vi "CreateAPSxObject.vi"(0 "PGIType":enum16{"APSX_PGI_TYPE_1", "APSX_PGI_TYPE_2"}(ring), 5 "DeviceNumber":i32, 7 "PGIChannel":i32, 9 "AsicName":string, 11 "error in (no error)":errorcluster caption="错误输入（无错误）") -> (4 "hASIC":i32, 10 "Message":string, 15 "error out":errorcluster caption="错误输出")   [LabVIEW 2018]
uses:
  APSx.dll/APSx.dll
panel:
  in  "hASIC IN":i32
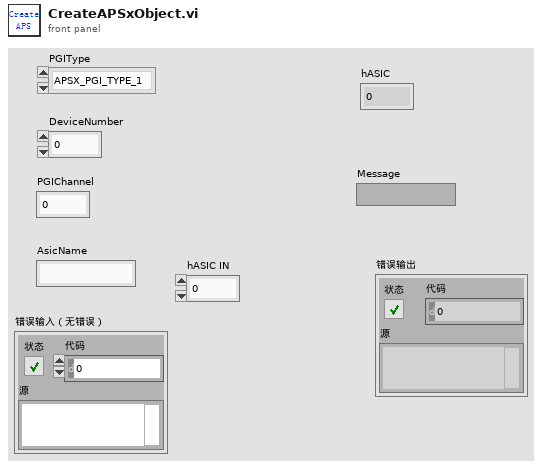
[diagram p1: front panel]
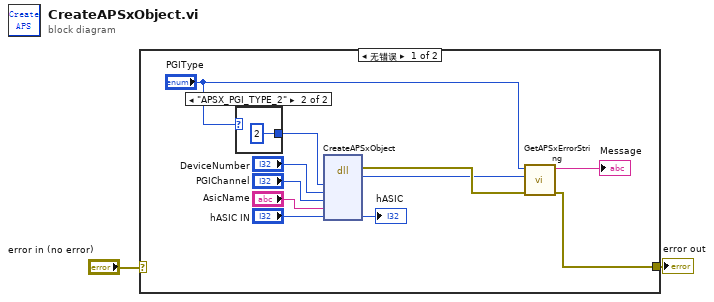
[diagram p0: block diagram]
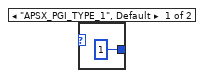
[diagram p2: hidden frame]
diagram:
  n1 = case shown="无错误" "error in (no error)" {
    selector: "error in (no error)" -> [_ w16]
    tunnel: [w4 w16] -> w1
    frame No Error {
      n2 = case shown="\"APSX_PGI_TYPE_2\"" "PGIType" {
        tunnel: [1 ("ComPort") 2 ("ComPort")] -> w8
        frame "APSX_PGI_TYPE_1", Default {
        }
        frame "APSX_PGI_TYPE_2" {
        }
      }
      n3 = dll-call lib="PTH2]abs D项目Feng恒隆项目Labview传感器对中台SourcesAPSx.dllAPSx.dll" fn="CreateAPSxObject"("PGIType"=w8, "DeviceNumber"="DeviceNumber", "PGIChannel"="PGIChannel", "AsicName"="AsicName", "hASIC"="hASIC IN") -> (error out=w7:errorcluster, "Code"=w5:i32, "hASIC"=→"hASIC":i32)  [unwired: 7 in, 1 out]
      n4 = call "GetAPSxErrorString.vi"("error in (no error)"=w7, "ErrorCode"=w5, "PGIType"="PGIType") -> ("error out"=w4:errorcluster, "Message"=→"Message":string)  [unwired: 7 in]
    }
    frame Error {
    }
  }
  "error out" <- w1
